vi "Sort Message[ ].vi"(8 "error in (no error)":errorcluster, 11 "Telegram Class in":refnum<class "Telegram Class.lvclass">) -> (0 "error out":errorcluster, 3 "Telegram Class out":refnum<class "Telegram Class.lvclass">)   [LabVIEW 2015, in "Telegram Library.lvlib" / "Telegram Class.lvclass"]
doc: "Created IvanLis by LabVIEW Portal\nProfile: http://labviewportal.org/memberlist.php?mode=viewprofile&u=987\neMail: IvanLisanov@gMail.com\nTelegram: https://t.me/IvanLis"
uses:
  Telegram Class.lvclass
  Telegram Class.lvclass/Telegram Class.ctl
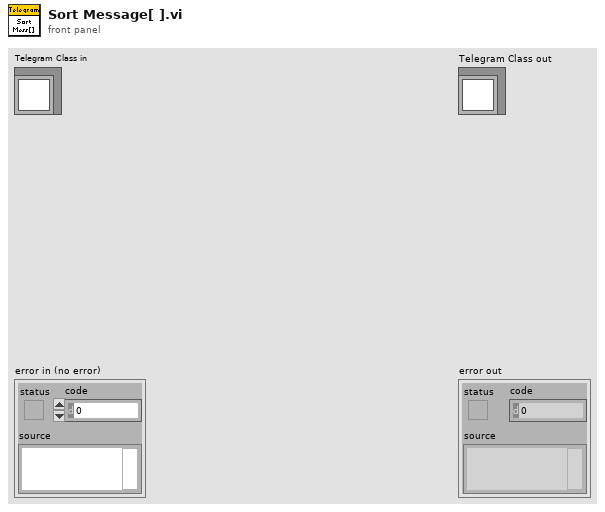
[diagram p1: front panel]
types:
  T1 = typedef "Telegram Library.lvlib/Message.ctl" = cluster{"id":i64, "chat_id":i64, "sender_user_id":i64, "date UTC":timestamp, "content_text":string}
  T2 = cluster{"date UTC":timestamp, "Message id[ ]":i64, "Message":T1}
  T3 = cluster{"date UTC":timestamp, "Message id[ ]":i64, "Message":T1}[]
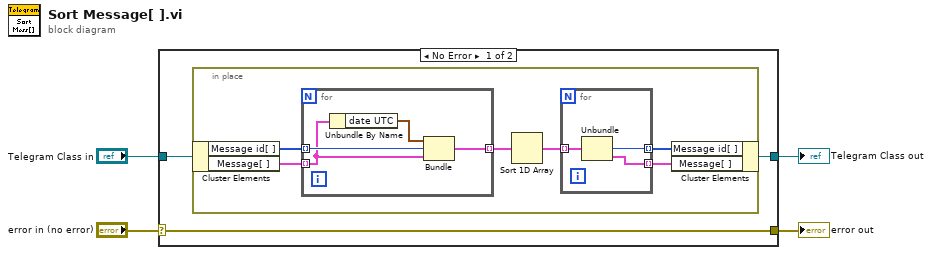
[diagram p0: block diagram]
diagram:
  n1 = case shown="No Error" "error in (no error)" {
    selector: "error in (no error)" -> [w7 w22]
    tunnel: [w7 w22] -> w3
    tunnel: [w5 w21] -> w1
    tunnel: "Telegram Class in" -> [w6 w21]
    frame No Error {
      n2 = in-place {
        n3 = in-place-cluster #1(w6) -> ("Message id[ ]"=w13:i64[], "Message[ ]"=w12:T1[])
        n4 = for {
          tunnel: w13 -> [w17] mode=indexing
          tunnel: w12 -> [w15] mode=indexing
          tunnel: [w16] -> w11 mode=indexing
          n5 = Unbundle By Name(w15) -> ("date UTC"=w14:timestamp)
          n6 = Bundle("date UTC"=w14, "Message id[ ]"=w17, "Message"=w15) -> (w16:T2)  [unwired: 1 in]
        }
        n7 = Sort 1D Array(array=w11) -> (sorted array=w8:T3)
        n8 = for {
          tunnel: w8 -> [w20] mode=indexing
          tunnel: [w19] -> w10 mode=indexing
          tunnel: [w18] -> w9 mode=indexing
          n9 = Unbundle(w20) -> ("Message id[ ]"=w19:i64, "Message"=w18:T1)  [unwired: 1 out]
        }
        n10 = in-place-cluster #1("Message id[ ]"=w10, "Message[ ]"=w9) -> (w5:refnum<class "Telegram Class.lvclass">)
      }
    }
    frame Error {
    }
  }
  "error out" <- w3
  "Telegram Class out" <- w1
